vi "(MAIN) __Mass Combat Sim.vi"() -> ()   [LabVIEW 2020]
uses:
  Utilities/Message_Log_Control.ctl
  MC5e Editor modes.ctl
  MC5e Squad_Manager_Modes.ctl
  MC5e Unit_Manager_Modes.ctl
  MC5e Gobal_Variables.vi
  <vilib>/Platform/browser.llb/Open URL in Default Browser (path).vi
panel:
  in  "Exit Program":bool
  out "date/time string":string="12/5/2020 8:11:19 PM : Aborted Program"
  in  "Tab Control":T1(tab)
  in  "Load Config Button":bool
  in  "Save Config Button":bool
  in  "Load Squads Button":bool
  in  "Save Squads Button":bool
  in  "Copy Squad Button":bool
  in  "Edit Squad Button":bool
  in  "Delete Squad Button":bool
  in  "New Squad Button":bool
  in  "Squad Summary":i32(listbox)
  in  "# to Move":u16=10 min=1
  in  "Remove ALL from Unit":bool
  in  "Add ALL to Unit":bool
  in  "Copy Unit Button":bool
  in  "Edit Unit Button":bool
  in  "Delete Unit Button":bool
  in  "New Unit Button":bool
  in  "Unit Summary":i32(listbox)
  in  "Load Units Button":bool
  in  "Save Units Button":bool
  in  "Squads in this Unit":i32(listbox)
  in  "Remove Squad from Unit":bool
  in  "Add Squad to Unit":bool
  in  "Available Squads":i32(listbox)
  in  "Open Debug Log":bool
  in  "Clear Log Button":bool
  out "Message Log":string="This message log will show logged messages and handled errors.  Copies of these messages are also stored in \nC:\\Users\\Public\\NI Logs\\Debug.log"
  out "last err code":i32
  out "last err source":string="0"
  out "Version":string
  out "Status Message":string="12/05/2020 08:11:19.588 PM -- Exit"
  # "Saves or loads settings"
  # "Mange Squads here then select on the next tab to build units."
  # "To add more available squads, use the \nSquads tab and copy or create new squads."
  # "To report bugs, please copy file C:\\Users\\Public\\NI Logs\\Debug.log and email to Steve Varga at varga.sm@pg.com"
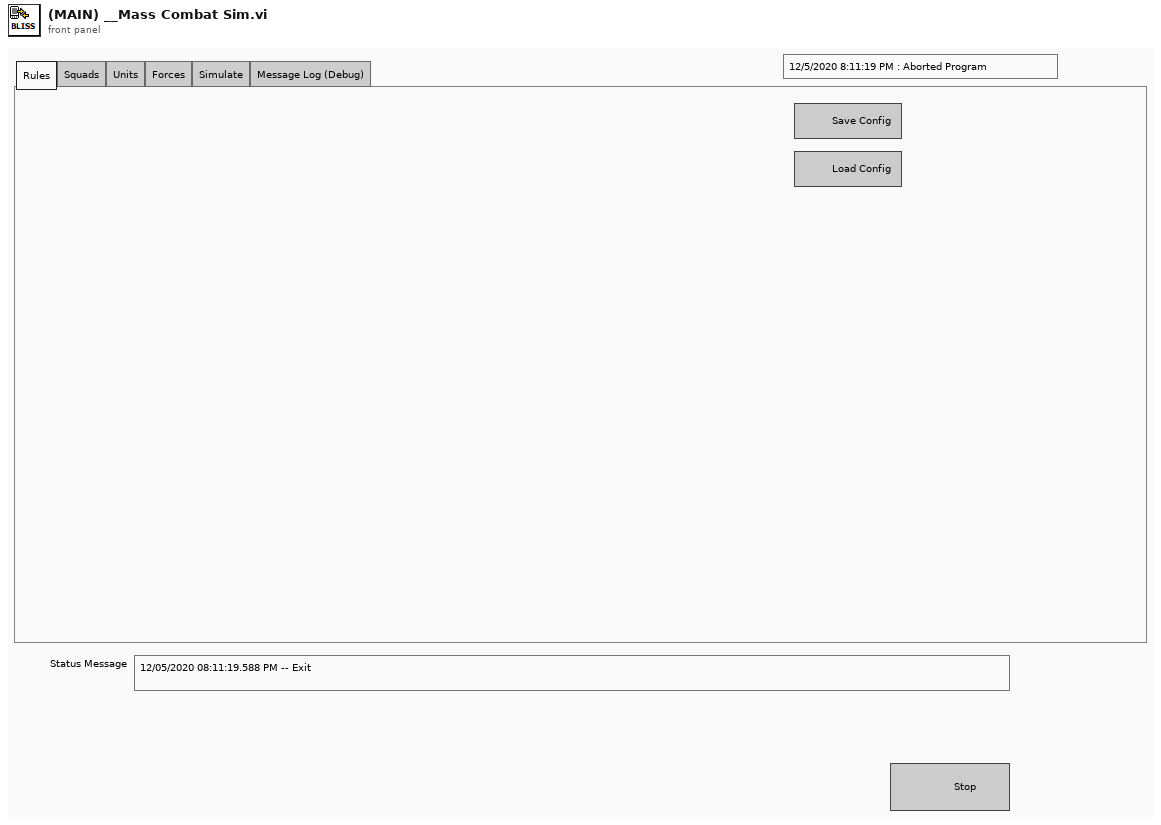
[diagram p1: front panel]
types:
  T1 = enum32{"Rules", "Squads", "Units", "Forces", "Simulate", "Message Log (Debug)"}
  T2 = typedef "Message_Log_Control.ctl" = enum16{"Add Entry", "Get Log", "Clear Log", "Clear First Error (unlatch)"}
  T3 = enum32{"invalid app kind", "Development System", "Run Time System", "Student Edition", "Embedded LabVIEW", "Evaluation", "Custom"}
  T4 = typedef "MC5e Command Q.ctl" = cluster{"Command":string, "Data String":string, "Variant":variant}
  T5 = typedef "MC5e Data_Parameters.ctl" = cluster{"Forces in Theater":T6[]}
  T6 = typedef "MC5e Force.ctl" = cluster{"Force Commander":string, "Units":T7[]}
  T7 = typedef "MC5e Unit.ctl" = cluster{"Unit Fatigue Level":enum16{"Not Fatigued", "Fatigued", "Seriously Fatigued"}, "Flying Unit":bool, "Mounted Unit":bool, "Defending from Stronghold":bool, "Difficult Terrain Types":T8, "Squads in Unit":T9[], "Unit Info":T11, "Range":i32, "BR":i32, "Speed":i32, "Morale":i32, "Current BR":i32, "Location":T12, "Capacity %":i32}
  T8 = typedef "MC5e Terrain types.ctl" = i32[]
  T9 = typedef "MC5e Squad_Info.ctl" = cluster{"Squad Name":string, "# Soldiers":u16, "Battle Rating":u16, "Flying":bool, "Mounted":bool, "Speed":u16, "Range":u16, "Morale":i32, "Max Endurance":u16, "Current Endurance":i32, "Size":T10, "Space Taken":u16, "Difficult Terrain":i32[], "CR":u16, "Special / Notes":string}
  T10 = typedef "MC5e Size_Categories.ctl" = enum16{"Tiny", "Small", "Medium", "Large", "Huge", "Gargantuan"}
  T11 = typedef "MC5e Unit Header.ctl" = cluster{"Unit Name":string, "Unit Commander":string, "Morale Mod":i32, "BR Mod":i32, "Defense Mod":i32, "Speed Mod":i32, "Unit Notes":string, "Attack Mod":i32, "Unit Wins+ Losses-":i32, "Commander Charisma Bonus":i32}
  T12 = typedef "Location.ctl" = cluster{"X coordinate":dbl, "Y coordinate":dbl}
  T13 = typedef "MC5e Editor modes.ctl" = enum16{"Add New", "Copy Selected", "Delete Selected", "Edit Selected"}
  T14 = typedef "LVRowAndColumnTypeDef.ctl" = cluster{"Row":i32, "Column":i32}
  T15 = typedef "MC5e Unit_Manager_Modes.ctl" = enum16{"Initialize", "Add Unit", "Delete Unit", "Get Unit", "Load Set", "Replace Unit"}
  T16 = typedef "MC5e Squad_Manager_Modes.ctl" = enum16{"Initialize", "Add Squad", "Delete Squad", "Get Squad", "Replace Squad", "Load Set"}
  T17 = enum8{"Enabled", "Disabled", "Disabled and Grayed Out"}
  T18 = enum16{"Only Controls", "Only Indicators", "Both (All)"}
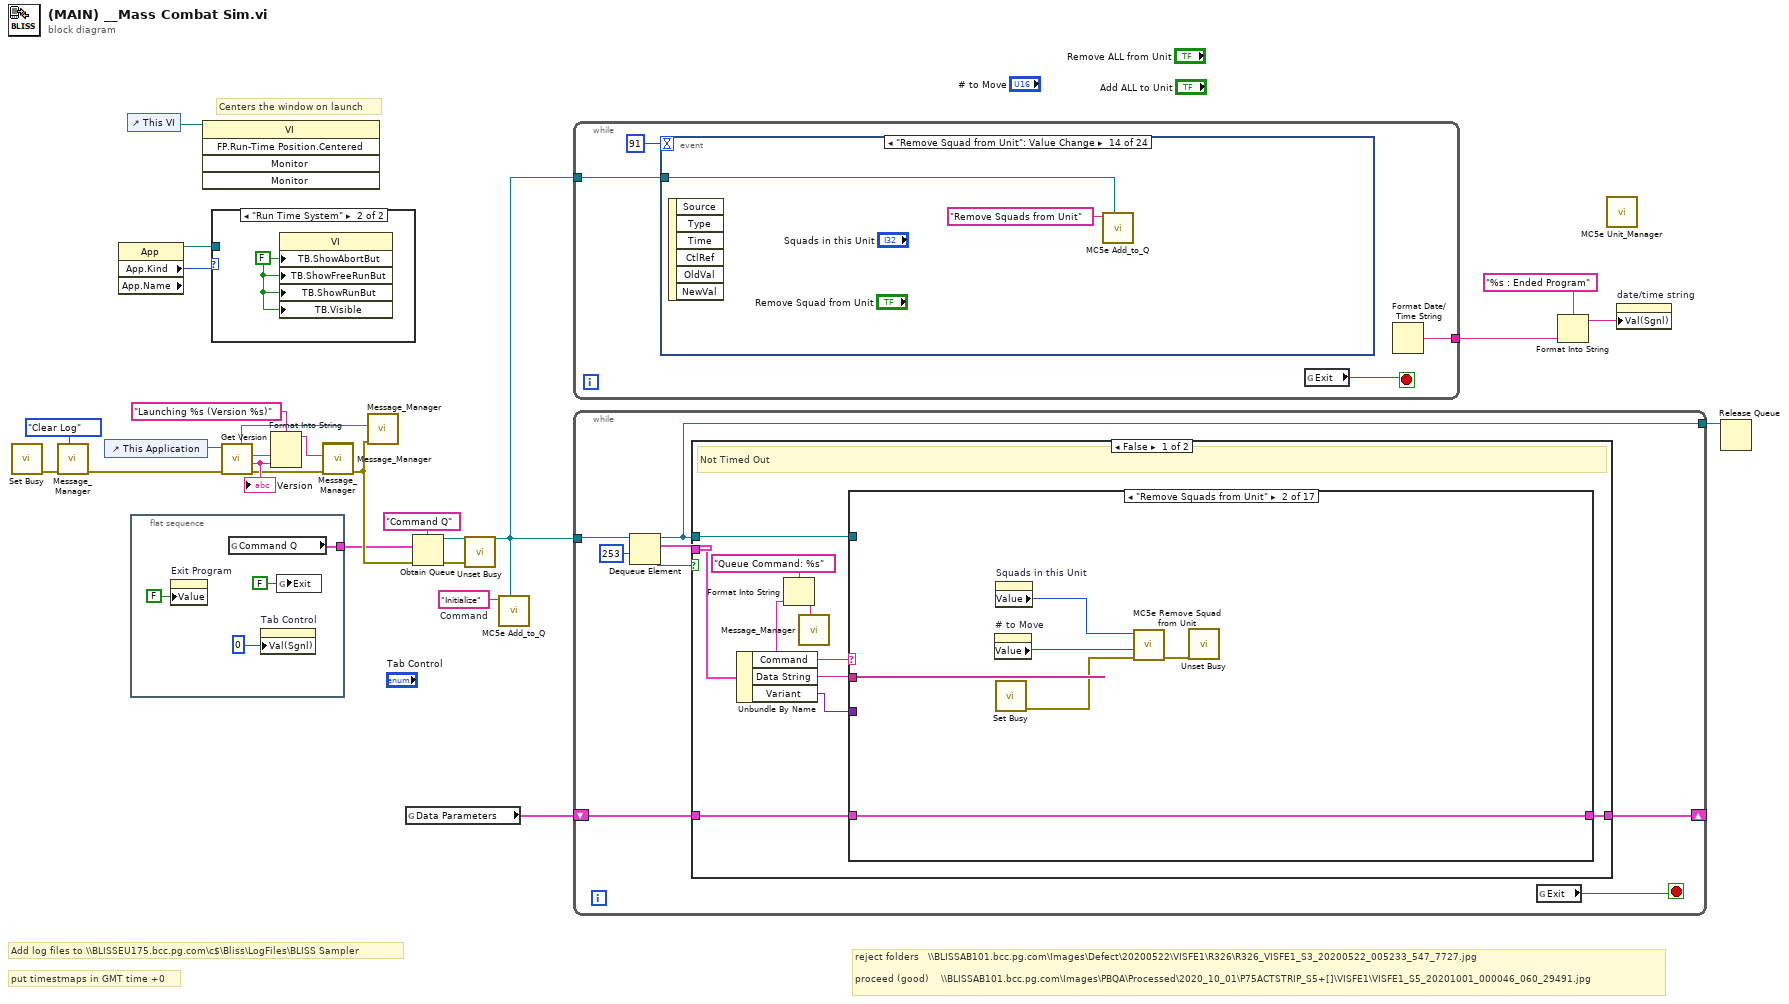
[diagram p0: block diagram]
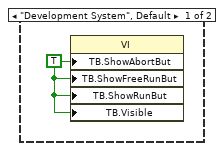
[diagram p2: hidden frame]
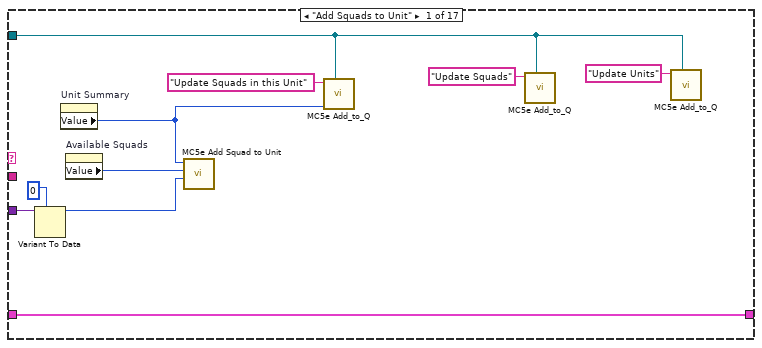
[diagram p3: hidden frame]
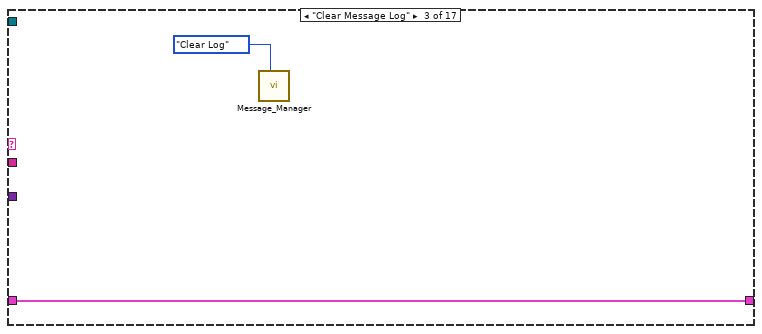
[diagram p4: hidden frame]
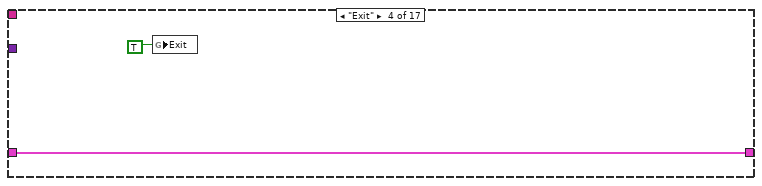
[diagram p5: hidden frame]
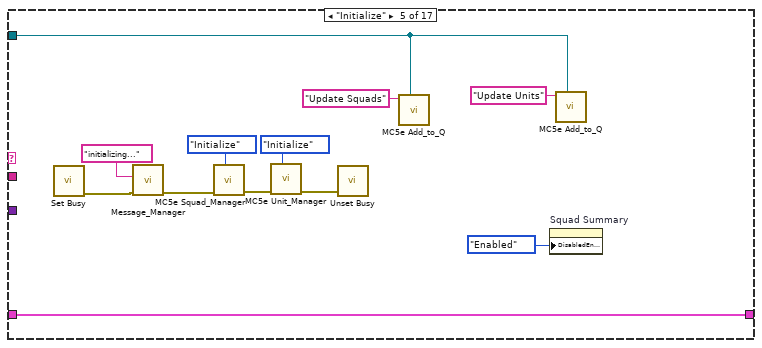
[diagram p6: hidden frame]
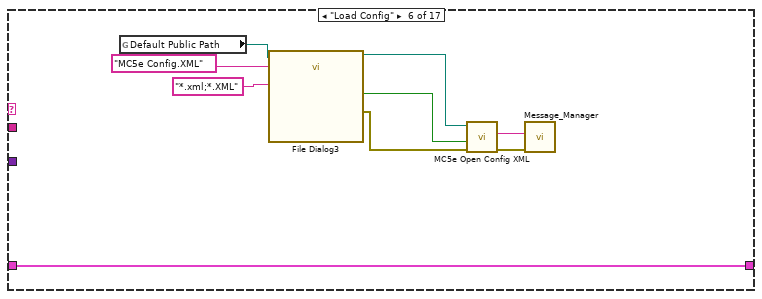
[diagram p7: hidden frame]
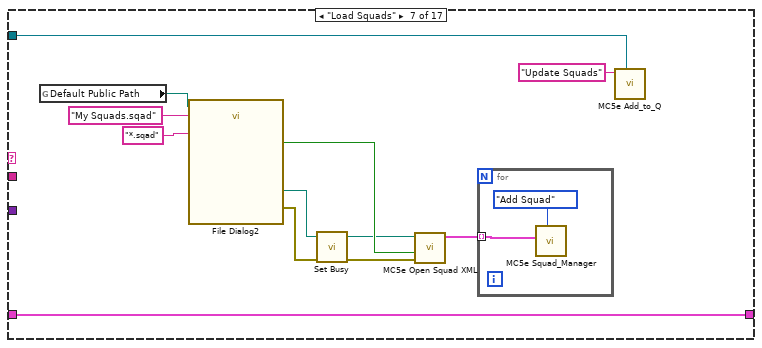
[diagram p8: hidden frame]
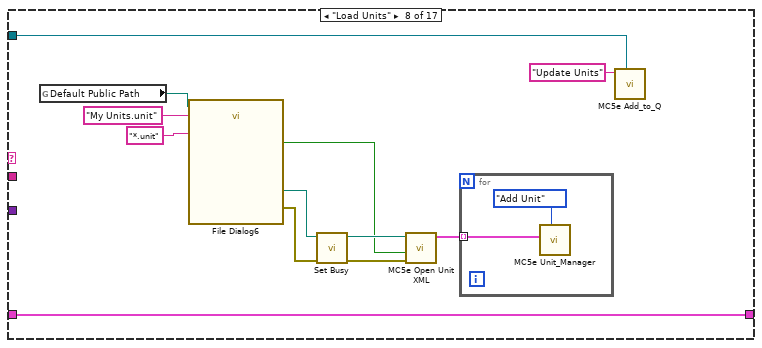
[diagram p9: hidden frame]
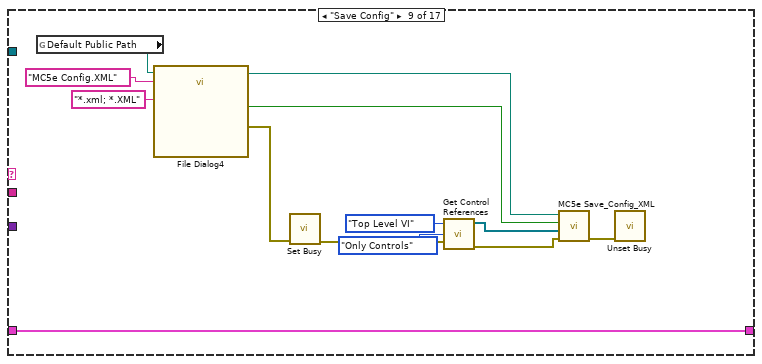
[diagram p10: hidden frame]
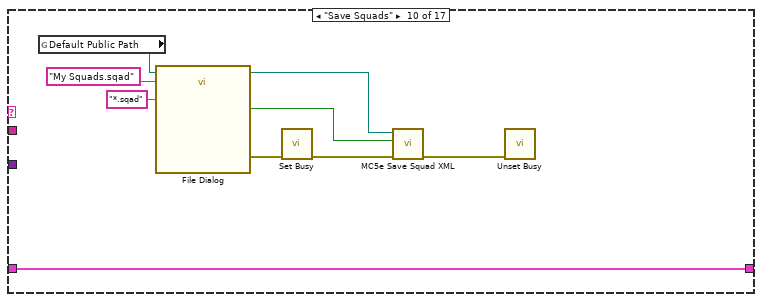
[diagram p11: hidden frame]
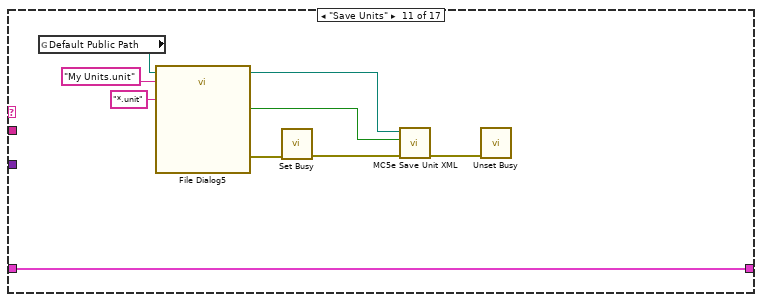
[diagram p12: hidden frame]
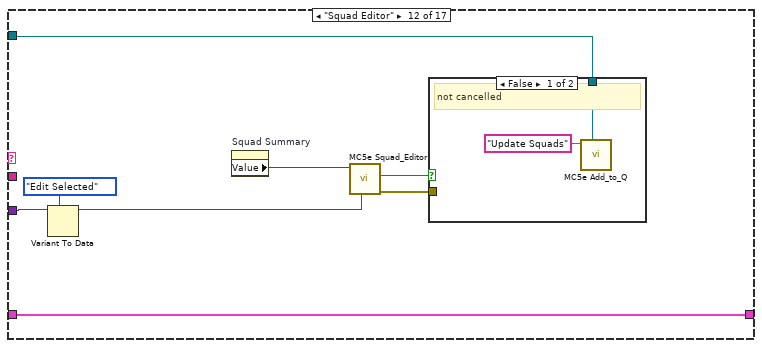
[diagram p13: hidden frame]
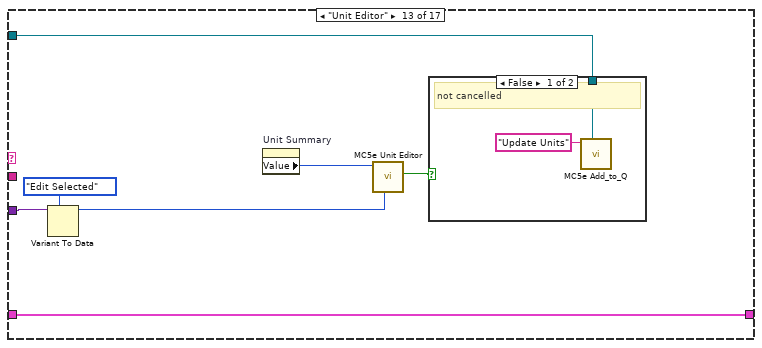
[diagram p15: hidden frame]
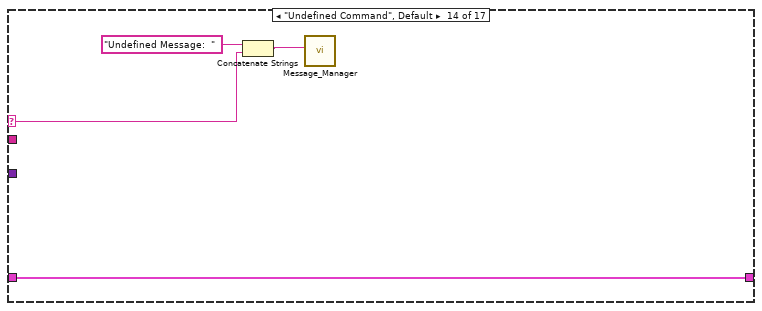
[diagram p17: hidden frame]
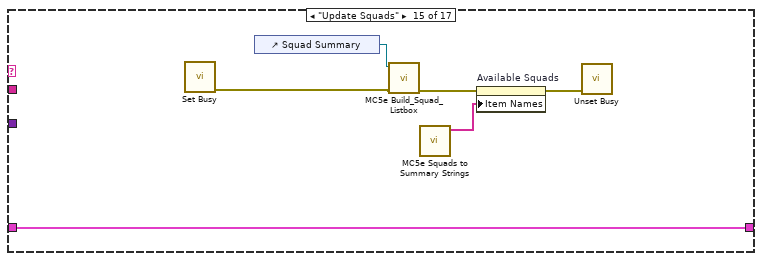
[diagram p18: hidden frame]
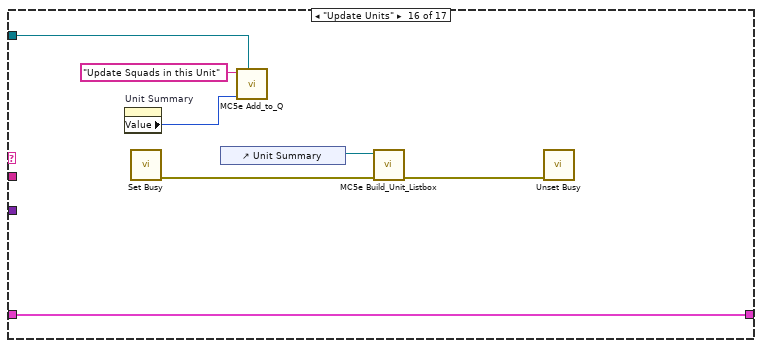
[diagram p19: hidden frame]
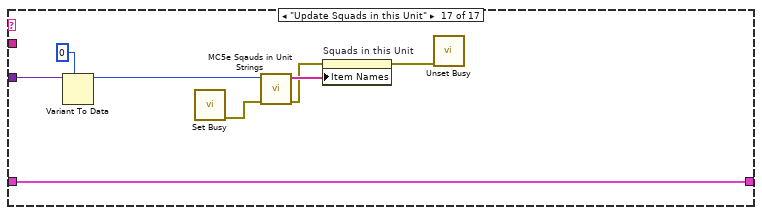
[diagram p20: hidden frame]
diagram:
  w22 = "Initialize"  # Command
  # "put timestmaps in GMT time +0"
  # "Add log files to \\\\BLISSEU175.bcc.pg.com\\c$\\Bliss\\LogFiles\\BLISS Sampler"
  # "Centers the window on launch"
  # "reject folders   \\\\BLISSAB101.bcc.pg.com\\Images\\Defect\\20200522\\VISFE1\\R326\\R326_VISFE1_S3_20200522_005233_547_7727.jpg\n\nproceed (good)    \\\\BLISSAB101.bcc.pg.com\\Images\\PBQA\\Processed\\2020_10_01\\P75ACTSTRIP_S5+[]\\VISFE1\\VISFE1_S5_20201001_000046_060_29491.jpg"
  n1 = call <vilib>:"Set Busy.vi"() -> ("error out"=w2:errorcluster)  [unwired: 10 in, 1 out]
  n2 = call "Message_Manager.vi"("Action (Add)"=Message_Log_Control."Clear Log", "error in"=w2) -> ("error out"=w4:errorcluster)  [unwired: 5 in, 4 out]
  n3 = control-ref of="This Application"() -> (w12:refnum<vi>)
  n4 = property class="App" props=["App.Kind", "App.Name"]() -> (reference out=w8:refnum<vi>, "App.Kind"=w9:T3)  [unwired: 2 in, 2 out]
  n5 = control-ref of="This VI"() -> (w18:refnum<vi>)
  n6 = flat-sequence {
    tunnel: [w28] -> w7
    frame #0 {
      n7 = property on="Exit Program" class="Bool (strict)"("Value"=FALSE ("Exit Program")) -> ()  [unwired: 2 in, 2 out]
      n8 = global read "MC5e Gobal_Variables.vi" "Command Q"() -> (w28:T4)
      n9 = property on="Tab Control" class="TabCtl (strict)"("Val(Sgnl)"=0) -> ()  [unwired: 2 in, 2 out]
      n10 = global write "MC5e Gobal_Variables.vi" "Exit"(FALSE ("Exit")) -> ()
    }
  }
  n11 = invoke class="VI" method="FP.Run-Time Position.Centered"(reference=w18) -> ()  [unwired: 4 in, 5 out]
  n12 = case shown="\"Run Time System\"" w9 {
    tunnel: w8 -> [_ _]
    frame "Development System", Default {
      w29 = TRUE ("Tool Bar:Show Abort Button")
      n13 = property class="VI"("TB.ShowAbortBut"=w29, "TB.ShowFreeRunBut"=w29, "TB.ShowRunBut"=w29, "TB.Visible"=w29) -> ()  [unwired: 2 in, 2 out]
    }
    frame "Run Time System" {
      w30 = FALSE ("Tool Bar:Show Abort Button")
      n14 = property class="VI"("TB.ShowAbortBut"=w30, "TB.ShowFreeRunBut"=w30, "TB.ShowRunBut"=w30, "TB.Visible"=w30) -> ()  [unwired: 2 in, 2 out]
    }
  }
  n15 = call "Get Version.vi"("Application Ref"=w12, "error in (no error)"=w4) -> ("Run Time info"=w11:string, "Name"=w16:string, "Version"=w15:string, "error out"=w14:errorcluster)  [unwired: 2 in, 1 out]
  "Version" <- w15
  n16 = Format Into String(format string="Launching %s (Version %s)", w16, w15) -> (resulting string=w13:string)  [unwired: 2 in, 1 out]
  n17 = call "Message_Manager.vi"() -> ()  [unwired: 7 in, 5 out]
  n18 = call "Message_Manager.vi"("error in"=w14, "New Entry"=w13) -> ("error out"=w10:errorcluster)  [unwired: 5 in, 4 out]
  n19 = call "Message_Manager.vi"("error in"=w10, "New Entry"=w11) -> ()  [unwired: 5 in, 5 out]
  n20 = global read "MC5e Gobal_Variables.vi" "Data Parameters"() -> (w5:T5)
  n21 = Obtain Queue(name (unnamed)="Command Q", element data type=w7, error in (no error)=w10) -> (queue out=w6:refnum<queue>, error out=w1:errorcluster)  [unwired: 2 in, 1 out]
  n22 = call <vilib>:"Unset Busy.vi"("error in (no error)"=w1) -> ()  [unwired: 10 in, 1 out]
  n23 = call "MC5e Add_to_Q.vi"("queue"=w6, "Command"=w22) -> ()  [unwired: 9 in, 1 out]
  n24 = while {
    tunnel: w6 -> [w34]
    tunnel: [w31] -> w19
    stop <- w33 stop-if-true
    n25 = event shown="[13] \"Remove Squad from Unit\": Value Change" {
      selector: _ -> [_ _ _ _ _ _ _ _ _ _ _ _ _ _ _ _ _ _ _ _ _ _ _ _]
      dyn-events: _ -> [_ _ _ _ _ _ _ _ _ _ _ _ _ _ _ _ _ _ _ _ _ _ _ _]
      timeout: 91 -> [_ _ _ _ _ _ _ _ _ _ _ _ _ _ _ _ _ _ _ _ _ _ _ _]
      tunnel: w34 -> [_ _ w43 w45 w47 _ w53 _ w68 w71 w76 w78 w80 w82 w85 w89 w90 w93 w96 w99 w101 w103 w106 w109]
      event Timeout {
        n26 = event-data() -> ()  [unwired: 1 in, 3 out]
        n27 = Format Date/Time String() -> (date/time string=→"date/time string":string)  [unwired: 3 in]
        n28 = call "Message_Manager.vi"("Action (Add)"=Message_Log_Control."Get Log") -> ("Last Err"=w37:cluster{"code":i32, "source":string}, "Last Message"=→"Status Message":string, "Message Log"=→"Message Log":string)  [unwired: 6 in, 2 out]
        n29 = Unbundle(w37) -> ("code"=→"last err code":i32, "source"=→"last err source":string)
      }
      event "Open Debug Log": Value Change {
        n30 = event-data() -> ()  [unwired: 1 in, 6 out]
        n31 = call-poly <vilib>:"Open URL in Default Browser.vi"("path"=path "C:/Users/Public/NI Logs/Debug.log") -> ()  [unwired: 5 in, 2 out]
      }
      event "Clear Log Button": Value Change {
        n32 = event-data() -> ()  [unwired: 1 in, 6 out]
        n33 = call "MC5e Add_to_Q.vi"("queue"=w43, "Command"="Clear Message Log") -> ()  [unwired: 9 in, 1 out]
      }
      event "Save Config Button": Value Change {
        n34 = event-data() -> ()  [unwired: 1 in, 6 out]
        n35 = call "MC5e Add_to_Q.vi"("queue"=w45, "Command"="Save Config") -> ()  [unwired: 9 in, 1 out]
      }
      event "Load Config Button": Value Change {
        n36 = event-data() -> ()  [unwired: 1 in, 6 out]
        n37 = call "MC5e Add_to_Q.vi"("queue"=w47, "Command"="Load Config") -> ()  [unwired: 9 in, 1 out]
      }
      event "Exit Program": Value Change {
        # "Exit function\njumps to the\nfront of the Q"
        n38 = event-data() -> ()  [unwired: 1 in, 5 out]
        n39 = call "MC5e Add_to_Q.vi"("Priority"=TRUE, "Command"="Exit") -> ()  [unwired: 9 in, 1 out]
      }
      event Panel Close? {
        n40 = event-data() -> ()  [unwired: 1 in, 4 out]
        n41 = Two Button Dialog(message="Are you sure you\nwant to exit?", 2:"Yes" ("T button name (\"OK\")")) -> (T button?=w52:bool)  [unwired: 1 in]
        n42 = case shown="True" w52 {
          tunnel: w53 -> [_ _]
          tunnel: [TRUE _] -> w51
          frame False {
          }
          frame True {
            n43 = call "MC5e Add_to_Q.vi"("Priority"=TRUE, "Command"="Exit") -> ()  [unwired: 9 in, 1 out]
          }
        }
        n44 = event-data("Discard?"=w51) -> ()  [unwired: 1 in, 1 out]
      }
      event "Squad Summary": Value Change {
        n45 = event-data() -> ()  [unwired: 1 in, 6 out]
        n46 = Format Into String(format string="squad selected %d", "Squad Summary") -> (resulting string=w61:string, error out=w60:errorcluster)  [unwired: 2 in]
        n47 = call "Message_Manager.vi"("error in"=w60, "New Entry"=w61) -> ()  [unwired: 5 in, 5 out]
      }
      event "Squad Summary": Double Click {
        n48 = event-data() -> ()  [unwired: 1 in, 8 out]
        n49 = property on="Squad Summary" class="MCListbox (strict)"() -> ("SelectedCell"=w65:T14, "Label.Text"=w63:string)  [unwired: 2 in, 2 out]
        n50 = Unbundle By Name(w65) -> ("Row"=w64:i32)
        n51 = property on="Squad Summary" class="MCListbox (strict)"("Value"=w64) -> ()  [unwired: 2 in, 2 out]
        n52 = call "MC5e Add_to_Q.vi"("queue"=w68, "Variant"=MC5e_Editor_modes."Edit Selected" ("Mode"), "Data"=w63, "Command"="Squad Editor") -> ()  [unwired: 7 in, 1 out]
      }
      event "Unit Summary": Value Change {
        n53 = event-data() -> ()  [unwired: 1 in, 6 out]
        n54 = Format Into String(format string="unit selected %d", "Unit Summary") -> (resulting string=w73:string, error out=w72:errorcluster)  [unwired: 2 in]
        n55 = call "Message_Manager.vi"("error in"=w72, "New Entry"=w73) -> ()  [unwired: 5 in, 5 out]
        n56 = call "MC5e Add_to_Q.vi"("queue"=w71, "Variant"="Unit Summary", "Command"="Update Squads in this Unit") -> ()  [unwired: 8 in, 1 out]
      }
      event "Save Squads Button": Value Change {
        n57 = event-data() -> ()  [unwired: 1 in, 6 out]
        n58 = call "MC5e Add_to_Q.vi"("queue"=w76, "Command"="Save Squads") -> ()  [unwired: 9 in, 1 out]
      }
      event "Load Squads Button": Value Change {
        n59 = event-data() -> ()  [unwired: 1 in, 6 out]
        n60 = call "MC5e Add_to_Q.vi"("queue"=w78, "Command"="Load Squads") -> ()  [unwired: 9 in, 1 out]
      }
      event "Add Squad to Unit": Value Change {
        n61 = event-data() -> ()  [unwired: 1 in, 6 out]
        n62 = property on="# to Move" class="DigNum (strict)"() -> ("Value"=w79:u16)  [unwired: 2 in, 2 out]
        n63 = call "MC5e Add_to_Q.vi"("queue"=w80, "Variant"=w79, "Command"="Add Squads to Unit") -> ()  [unwired: 8 in, 1 out]
      }
      event "Remove Squad from Unit": Value Change {
        n64 = event-data() -> ()  [unwired: 1 in, 6 out]
        n65 = call "MC5e Add_to_Q.vi"("queue"=w82, "Command"="Remove Squads from Unit") -> ()  [unwired: 9 in, 1 out]
      }
      event "New Squad Button": Value Change {
        n66 = event-data() -> ()  [unwired: 1 in, 6 out]
        n67 = call "MC5e Add_to_Q.vi"("queue"=w85, "Variant"=MC5e_Editor_modes."Add New" ("Mode"), "Command"="Squad Editor") -> ()  [unwired: 8 in, 1 out]
      }
      event "New Unit Button": Value Change {
        n68 = event-data() -> ()  [unwired: 1 in, 6 out]
        n69 = call "MC5e Add_to_Q.vi"("queue"=w89, "Variant"=MC5e_Editor_modes."Add New" ("Mode"), "Command"="Unit Editor") -> ()  [unwired: 8 in, 1 out]
      }
      event "Edit Unit Button": Value Change {
        n70 = event-data() -> ()  [unwired: 1 in, 6 out]
        n71 = call "MC5e Add_to_Q.vi"("queue"=w90, "Variant"=MC5e_Editor_modes."Edit Selected" ("Mode"), "Command"="Unit Editor") -> ()  [unwired: 8 in, 1 out]
      }
      event "Copy Unit Button": Value Change {
        n72 = event-data() -> ()  [unwired: 1 in, 6 out]
        n73 = call "MC5e Add_to_Q.vi"("queue"=w93, "Variant"=MC5e_Editor_modes."Copy Selected" ("Mode"), "Command"="Unit Editor") -> ()  [unwired: 8 in, 1 out]
      }
      event "Delete Unit Button": Value Change {
        n74 = event-data() -> ()  [unwired: 1 in, 6 out]
        n75 = call "MC5e Add_to_Q.vi"("queue"=w96, "Variant"=MC5e_Editor_modes."Delete Selected" ("Mode"), "Command"="Unit Editor") -> ()  [unwired: 8 in, 1 out]
      }
      event "Save Units Button": Value Change {
        n76 = event-data() -> ()  [unwired: 1 in, 6 out]
        n77 = call "MC5e Add_to_Q.vi"("queue"=w99, "Command"="Save Units") -> ()  [unwired: 9 in, 1 out]
      }
      event "Load Units Button": Value Change {
        n78 = event-data() -> ()  [unwired: 1 in, 6 out]
        n79 = call "MC5e Add_to_Q.vi"("queue"=w101, "Command"="Load Units") -> ()  [unwired: 9 in, 1 out]
      }
      event "Copy Squad Button": Value Change {
        n80 = event-data() -> ()  [unwired: 1 in, 6 out]
        n81 = call "MC5e Add_to_Q.vi"("queue"=w103, "Variant"=MC5e_Editor_modes."Copy Selected" ("Mode"), "Command"="Squad Editor") -> ()  [unwired: 8 in, 1 out]
      }
      event "Delete Squad Button": Value Change {
        n82 = event-data() -> ()  [unwired: 1 in, 6 out]
        n83 = call "MC5e Add_to_Q.vi"("queue"=w106, "Variant"=MC5e_Editor_modes."Delete Selected" ("Mode"), "Command"="Squad Editor") -> ()  [unwired: 8 in, 1 out]
      }
      event "Edit Squad Button": Value Change {
        n84 = event-data() -> ()  [unwired: 1 in, 6 out]
        n85 = call "MC5e Add_to_Q.vi"("queue"=w109, "Variant"=MC5e_Editor_modes."Edit Selected" ("Mode"), "Command"="Squad Editor") -> ()  [unwired: 8 in, 1 out]
      }
    }
    n86 = global read "MC5e Gobal_Variables.vi" "Exit"() -> (w33:bool)
    n87 = Format Date/Time String() -> (date/time string=w31:string)  [unwired: 3 in]
  }
  n88 = while {
    tunnel: w6 -> [w117]
    tunnel: [w114] -> w23
    shift-right: [w112] -> _
    shift-left: w5 -> [w113]
    stop <- w116 stop-if-true
    n89 = Dequeue Element(queue=w117, timeout in ms (-1)=253) -> (queue out=w114:refnum<queue>, element=w118:T4, timed out?=w119:bool)  [unwired: 1 in, 1 out]
    n90 = case shown="False" w119 {
      tunnel: w118 -> [w121 _]
      tunnel: w114 -> [w128 _]
      tunnel: w113 -> [w123 w270]
      tunnel: [w122 w270] -> w112
      frame False {
        # "Not Timed Out"
        n91 = Unbundle By Name(w121) -> ("Command"=w120:string, "Data String"=w127:string, "Variant"=w126:variant)
        n92 = Format Into String(format string="Queue Command: %s", w120) -> (resulting string=w124:string)  [unwired: 2 in, 1 out]
        n93 = call "Message_Manager.vi"("New Entry"=w124) -> ()  [unwired: 6 in, 5 out]
        n94 = case shown="\"Remove Squads from Unit\"" w120 {
          selector: w120 -> [_ _ _ _ _ _ _ _ _ _ _ _ _ w247 _ _ _]
          tunnel: w128 -> [w129 _ _ _ w148 _ w178 w191 _ _ _ w227 w239 _ _ w255 _]
          tunnel: w127 -> [_ _ _ _ _ _ _ _ _ _ _ _ _ _ _ _ _]
          tunnel: w126 -> [w137 _ _ _ _ _ _ _ _ _ _ w232 w241 _ _ _ w266]
          tunnel: w123 -> [w138 w143 w144 w146 w158 w168 w177 w190 w205 w213 w222 w233 w242 w245 w254 w261 w262]
          tunnel: [w138 w143 w144 w146 w158 w168 w177 w190 w205 w213 w222 w233 w242 w245 w254 w261 w262] -> w122
          frame "Add Squads to Unit" {
            n95 = Variant To Data(type=u16 0, Variant=w137) -> (data=w134:u16)  [unwired: 1 in, 1 out]
            n96 = property on="Unit Summary" class="MCListbox (strict)"() -> ("Value"=w132:i32)  [unwired: 2 in, 2 out]
            n97 = property on="Available Squads" class="LstBox (strict)"() -> ("Value"=w135:i32)  [unwired: 2 in, 2 out]
            n98 = call "MC5e Add Squad to Unit.vi"("# to add"=w134, "Squad Index"=w135, "Unit Index"=w132) -> ()  [unwired: 9 in]
            n99 = call "MC5e Add_to_Q.vi"("queue"=w129, "Variant"=w132, "Command"="Update Squads in this Unit") -> ()  [unwired: 8 in, 1 out]
            n100 = call "MC5e Add_to_Q.vi"("queue"=w129, "Command"="Update Squads") -> ()  [unwired: 9 in, 1 out]
            n101 = call "MC5e Add_to_Q.vi"("queue"=w129, "Command"="Update Units") -> ()  [unwired: 9 in, 1 out]
          }
          frame "Remove Squads from Unit" {
            n102 = property on="# to Move" class="DigNum (strict)"() -> ("Value"=w142:u16)  [unwired: 2 in, 2 out]
            n103 = property on="Squads in this Unit" class="LstBox (strict)"() -> ("Value"=w141:i32)  [unwired: 2 in, 2 out]
            n104 = call <vilib>:"Set Busy.vi"() -> ("error out"=w140:errorcluster)  [unwired: 10 in, 1 out]
            n105 = call "MC5e Remove Squad from Unit.vi"("error in"=w140, "# to remove"=w142, "Unit Index"=w141) -> ("error out"=w139:errorcluster)  [unwired: 8 in]
            n106 = call <vilib>:"Unset Busy.vi"("error in (no error)"=w139) -> ()  [unwired: 10 in, 1 out]
          }
          frame "Clear Message Log" {
            n107 = call "Message_Manager.vi"("Action (Add)"=Message_Log_Control."Clear Log") -> ()  [unwired: 6 in, 5 out]
          }
          frame "Exit" {
            n108 = global write "MC5e Gobal_Variables.vi" "Exit"(TRUE ("Exit")) -> ()
          }
          frame "Initialize" {
            n109 = call <vilib>:"Set Busy.vi"() -> ("error out"=w153:errorcluster)  [unwired: 10 in, 1 out]
            n110 = call "Message_Manager.vi"("error in"=w153, "New Entry"="initializing...") -> ("error out"=w155:errorcluster)  [unwired: 5 in, 4 out]
            n111 = call "MC5e Squad_Manager.vi"("Mode (Get)"=MC5e_Squad_Manager_Modes."Initialize" ("Mode"), "error in"=w155) -> ("error out"=w152:errorcluster)  [unwired: 6 in, 3 out]
            n112 = call "MC5e Unit_Manager.vi"("Mode (Get)"=MC5e_Unit_Manager_Modes."Initialize", "error in"=w152) -> ("error out"=w151:errorcluster)  [unwired: 6 in, 3 out]
            n113 = call <vilib>:"Unset Busy.vi"("error in (no error)"=w151) -> ()  [unwired: 10 in, 1 out]
            n114 = call "MC5e Add_to_Q.vi"("queue"=w148, "Command"="Update Squads") -> ()  [unwired: 9 in, 1 out]
            n115 = property on="Squad Summary" class="MCListbox (strict)"("DisabledEnum"=T17."Enabled" ("Disabled")) -> ()  [unwired: 2 in, 2 out]
            n116 = call "MC5e Add_to_Q.vi"("queue"=w148, "Command"="Update Units") -> ()  [unwired: 9 in, 1 out]
          }
          frame "Load Config" {
            n117 = global read "MC5e Gobal_Variables.vi" "Default Public Path"() -> (w166:path)
            n118 = call "File Dialog3"("start path"=w166, "default name"="MC5e Config.XML", "pattern (all files)"="*.xml;*.XML") -> ("selected path"=w163:path, "cancelled"=w162:bool, "error out"=w161:errorcluster)  [unwired: 9 in, 1 out]
            n119 = call "MC5e Open Config XML.vi"("error in"=w161, "Cancelled?"=w162, "selected path"=w163) -> ("error out"=w164:errorcluster, "SHA256 Hash of Controls"=w160:string)  [unwired: 6 in, 1 out]
            n120 = call "Message_Manager.vi"("error in"=w164, "New Entry"=w160) -> ()  [unwired: 5 in, 5 out]
          }
          frame "Load Squads" {
            n121 = global read "MC5e Gobal_Variables.vi" "Default Public Path"() -> (w173:path)
            n122 = call "File Dialog2"("start path"=w173, "default name"="My Squads.sqad", "pattern (all files)"="*.sqad") -> ("selected path"=w170:path, "cancelled"=w172:bool, "error out"=w171:errorcluster)  [unwired: 9 in, 1 out]
            n123 = call <vilib>:"Set Busy.vi"("error in (no error)"=w171) -> ("error out"=w169:errorcluster)  [unwired: 9 in, 1 out]
            n124 = call "MC5e Open Squad XML.vi"("error in"=w169, "Cancelled?"=w172, "selected path"=w170) -> ("Squad Array"=w176:T9[])  [unwired: 7 in, 1 out]
            n125 = for {
              tunnel: w176 -> [w180] mode=indexing
              n126 = call "MC5e Squad_Manager.vi"("Mode (Get)"=MC5e_Squad_Manager_Modes."Add Squad", "Squad in (add/replace)"=w180) -> ()  [unwired: 6 in, 4 out]
            }
            n127 = call "MC5e Add_to_Q.vi"("queue"=w178, "Command"="Update Squads") -> ()  [unwired: 9 in, 1 out]
          }
          frame "Load Units" {
            n128 = global read "MC5e Gobal_Variables.vi" "Default Public Path"() -> (w187:path)
            n129 = call "File Dialog6"("start path"=w187, "default name"="My Units.unit", "pattern (all files)"="*.unit") -> ("selected path"=w185:path, "cancelled"=w184:bool, "error out"=w186:errorcluster)  [unwired: 9 in, 1 out]
            n130 = call <vilib>:"Set Busy.vi"("error in (no error)"=w186) -> ("error out"=w183:errorcluster)  [unwired: 9 in, 1 out]
            n131 = call "MC5e Open Unit XML.vi"("error in"=w183, "Cancelled?"=w184, "selected path"=w185) -> ("Unit Array"=w182:T7[])  [unwired: 7 in, 1 out]
            n132 = for {
              tunnel: w182 -> [w194] mode=indexing
              n133 = call "MC5e Unit_Manager.vi"("Mode (Get)"=MC5e_Unit_Manager_Modes."Add Unit", "Unit In (Add/Replace)"=w194) -> ()  [unwired: 6 in, 4 out]
            }
            n134 = call "MC5e Add_to_Q.vi"("queue"=w191, "Command"="Update Units") -> ()  [unwired: 9 in, 1 out]
          }
          frame "Save Config" {
            n135 = global read "MC5e Gobal_Variables.vi" "Default Public Path"() -> (w201:path)
            n136 = call "File Dialog4"("start path"=w201, "default name"="MC5e Config.XML", "pattern (all files)"="*.xml; *.XML") -> ("selected path"=w200:path, "cancelled"=w196:bool, "error out"=w198:errorcluster)  [unwired: 9 in, 1 out]
            n137 = call <vilib>:"Set Busy.vi"("error in (no error)"=w198) -> ("error out"=w204:errorcluster)  [unwired: 9 in, 1 out]
            n138 = call "Get Control References.vi"("error in"=w204, "Types"=T18."Only Controls", "Mode (Top Level)"=enum16{"Top Level VI", "This VI's caller"}."Top Level VI") -> ("error out"=w197:errorcluster, "References[]"=w195:refnum<vi>[])  [unwired: 1 in, 3 out]
            n139 = call "MC5e Save_Config_XML.vi"("error In"=w197, "Control References[]"=w195, "Cancelled?"=w196, "selected path"=w200) -> ("error out"=w199:errorcluster)  [unwired: 7 in]
            n140 = call <vilib>:"Unset Busy.vi"("error in (no error)"=w199) -> ()  [unwired: 10 in, 1 out]
          }
          frame "Save Squads" {
            n141 = global read "MC5e Gobal_Variables.vi" "Default Public Path"() -> (w214:path)
            n142 = call "File Dialog"("start path"=w214, "default name"="My Squads.sqad", "pattern (all files)"="*.sqad") -> ("selected path"=w209:path, "cancelled"=w208:bool, "error out"=w212:errorcluster)  [unwired: 9 in, 1 out]
            n143 = call <vilib>:"Set Busy.vi"("error in (no error)"=w212) -> ("error out"=w211:errorcluster)  [unwired: 9 in, 1 out]
            n144 = call "MC5e Save Squad XML.vi"("error in"=w211, "Cancelled?"=w208, "selected path"=w209) -> ("error out"=w210:errorcluster)  [unwired: 8 in]
            n145 = call <vilib>:"Unset Busy.vi"("error in (no error)"=w210) -> ()  [unwired: 10 in, 1 out]
          }
          frame "Save Units" {
            n146 = global read "MC5e Gobal_Variables.vi" "Default Public Path"() -> (w223:path)
            n147 = call "File Dialog5"("start path"=w223, "default name"="My Units.unit", "pattern (all files)"="*.unit") -> ("selected path"=w218:path, "cancelled"=w217:bool, "error out"=w221:errorcluster)  [unwired: 9 in, 1 out]
            n148 = call <vilib>:"Set Busy.vi"("error in (no error)"=w221) -> ("error out"=w220:errorcluster)  [unwired: 9 in, 1 out]
            n149 = call "MC5e Save Unit XML.vi"("error in"=w220, "Cancelled?"=w217, "selected path"=w218) -> ("error out"=w219:errorcluster)  [unwired: 8 in]
            n150 = call <vilib>:"Unset Busy.vi"("error in (no error)"=w219) -> ()  [unwired: 10 in, 1 out]
          }
          frame "Squad Editor" {
            n151 = Variant To Data(type=MC5e_Editor_modes."Edit Selected" ("Mode"), Variant=w232) -> (data=w230:T13)  [unwired: 1 in, 1 out]
            n152 = property on="Squad Summary" class="MCListbox (strict)"() -> ("Value"=w226:i32)  [unwired: 2 in, 2 out]
            n153 = call "MC5e Squad_Editor.vi"("Mode"=w230, "index"=w226) -> ("error out"=w229:errorcluster, "Cancelled"=w228:bool)  [unwired: 8 in]
            n154 = case shown="False" w228 {
              tunnel: w229 -> [_ _]
              tunnel: w227 -> [w234 _]
              frame False {
                # "not cancelled"
                n155 = call "MC5e Add_to_Q.vi"("queue"=w234, "Command"="Update Squads") -> ()  [unwired: 9 in, 1 out]
              }
              frame True {
                # "cancelled"
              }
            }
          }
          frame "Unit Editor" {
            n156 = Variant To Data(type=MC5e_Editor_modes."Edit Selected" ("Mode"), Variant=w241) -> (data=w237:T13)  [unwired: 1 in, 1 out]
            n157 = property on="Unit Summary" class="MCListbox (strict)"() -> ("Value"=w238:i32)  [unwired: 2 in, 2 out]
            n158 = call "MC5e Unit Editor.vi"("Mode"=w237, "index"=w238) -> ("Cancelled"=w236:bool)  [unwired: 8 in, 1 out]
            n159 = case shown="False" w236 {
              tunnel: w239 -> [w243 _]
              frame False {
                # "not cancelled"
                n160 = call "MC5e Add_to_Q.vi"("queue"=w243, "Command"="Update Units") -> ()  [unwired: 9 in, 1 out]
              }
              frame True {
                # "cancelled"
              }
            }
          }
          frame "Undefined Command", Default {
            n161 = Concatenate Strings("Undefined Message:  " ("format string"), w247) -> (w246:string)
            n162 = call "Message_Manager.vi"("New Entry"=w246) -> ()  [unwired: 6 in, 5 out]
          }
          frame "Update Squads" {
            n163 = call <vilib>:"Set Busy.vi"() -> ("error out"=w253:errorcluster)  [unwired: 10 in, 1 out]
            n164 = control-ref of="Squad Summary"() -> (w249:refnum<vi>)
            n165 = call "MC5e Build_Squad_Listbox.vi"("error in (no error)"=w253, "Squad Summary Ref"=w249) -> ("error out"=w252:errorcluster)  [unwired: 9 in]
            n166 = call "MC5e Squads to Summary Strings.vi"() -> ("Squad Strings"=w250:string[])  [unwired: 11 in]
            n167 = property on="Available Squads" class="LstBox (strict)"(error in=w252, "Item Names"=w250) -> (error out=w251:errorcluster)  [unwired: 1 in, 1 out]
            n168 = call <vilib>:"Unset Busy.vi"("error in (no error)"=w251) -> ()  [unwired: 10 in, 1 out]
          }
          frame "Update Units" {
            n169 = property on="Unit Summary" class="MCListbox (strict)"() -> ("Value"=w256:i32)  [unwired: 2 in, 2 out]
            n170 = call <vilib>:"Set Busy.vi"() -> ("error out"=w260:errorcluster)  [unwired: 10 in, 1 out]
            n171 = control-ref of="Unit Summary"() -> (w259:refnum<vi>)
            n172 = call "MC5e Add_to_Q.vi"("queue"=w255, "Variant"=w256, "Command"="Update Squads in this Unit") -> ()  [unwired: 8 in, 1 out]
            n173 = call "MC5e Build_Unit_Listbox.vi"("error in (no error)"=w260, "Unit Multilist Ref"=w259) -> ("error out"=w258:errorcluster)  [unwired: 9 in]
            n174 = call <vilib>:"Unset Busy.vi"("error in (no error)"=w258) -> ()  [unwired: 10 in, 1 out]
          }
          frame "Update Squads in this Unit" {
            n175 = Variant To Data(type=0, Variant=w266) -> (data=w265:i32)  [unwired: 1 in, 1 out]
            n176 = call <vilib>:"Set Busy.vi"() -> ("error out"=w264:errorcluster)  [unwired: 10 in, 1 out]
            n177 = call "MC5e Sqauds in Unit Strings.vi"("error in"=w264, "Unit index"=w265) -> ("error out"=w263:errorcluster, "Squad Strings"=w269:string[])  [unwired: 8 in]
            n178 = property on="Squads in this Unit" class="LstBox (strict)"(error in=w263, "Item Names"=w269) -> (error out=w268:errorcluster)  [unwired: 1 in, 1 out]
            n179 = call <vilib>:"Unset Busy.vi"("error in (no error)"=w268) -> ()  [unwired: 10 in, 1 out]
          }
        }
      }
      frame True {
        # "Timed Out (nothing new)"
        n180 = call <vilib>:"Unset Busy.vi"() -> ()  [unwired: 11 in, 1 out]
      }
    }
    n181 = global read "MC5e Gobal_Variables.vi" "Exit"() -> (w116:bool)
  }
  n182 = Format Into String(format string="%s : Ended Program", w19) -> (resulting string=w21:string)  [unwired: 2 in, 1 out]
  n183 = call "MC5e Unit_Manager.vi"() -> ()  [unwired: 8 in, 4 out]
  n184 = property on="date/time string" class="Str"("Val(Sgnl)"=w21) -> ()  [unwired: 2 in, 2 out]
  n185 = Release Queue(queue=w23) -> ()  [unwired: 2 in, 3 out]
